vi "RESTORE USER TO DATABASE.vi"(10 "DATA IN":string[][](array[string]), 11 "REFERENCES":T1) -> ()   [LabVIEW 2019]
uses:
  Controls/References Cluster.ctl
  Controls/Custom Calendar/Custom Calendar.xctl
  Controls/Table Data Types/User Archive Data Type.ctl
  Controls/Table Data Types/User Data Type.ctl
  <vilib>/addons/database/Connection.llb/DB Tools Open Connec (String).vi
  <vilib>/addons/database/_DB Variant To Data/Database Variant To Data.xnode
  <vilib>/addons/database/NI_Database_API.lvlib
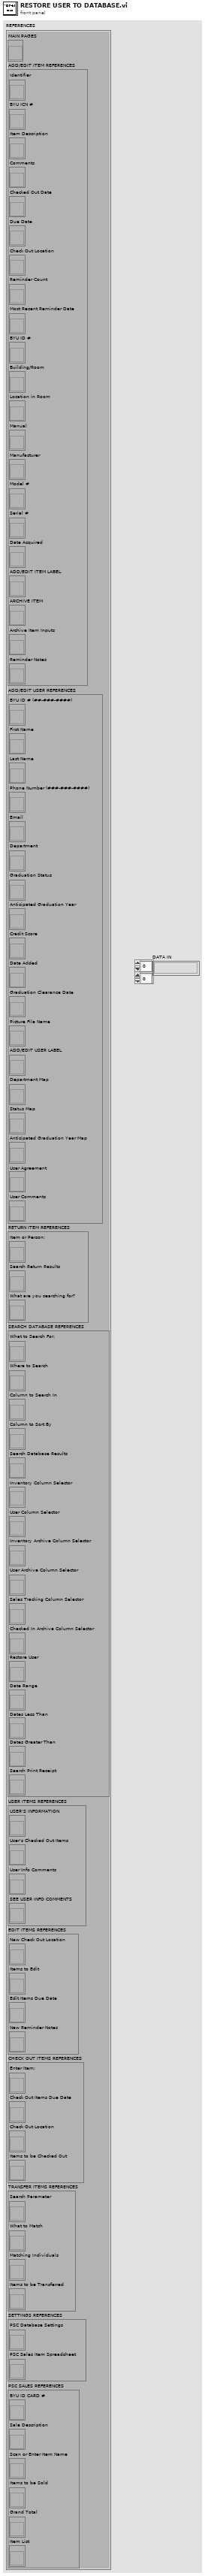
[diagram p1: front panel]
types:
  T1 = typedef "References Cluster.ctl" = cluster{"MAIN PAGES":refnum<vi>, "ADD/EDIT ITEM REFERENCES":cluster{"Identifier":refnum<vi>, "BYU ICN #":refnum<vi>, "Item Description":refnum<vi>, "Comments":refnum<vi>, "Checked Out Date":refnum<vi>, "Due Date":refnum<vi>, "Check Out Location":refnum<vi>, "Reminder Count":refnum<vi>, "Most Recent Reminder Date":refnum<vi>, "BYU ID #":refnum<vi>, "Building/Room":refnum<vi>, "Location in Room":refnum<vi>, "Manual":refnum<vi>, "Manufacturer":refnum<vi>, "Model #":refnum<vi>, "Serial #":refnum<vi>, "Date Acquired":refnum<vi>, "ADD/EDIT ITEM LABEL":refnum<vi>, "ARCHIVE ITEM":refnum<vi>, "Archive Item Inputs":refnum<vi>, "Reminder Notes":refnum<vi>}, "ADD/EDIT USER REFERENCES":cluster{"BYU ID # (##-###-####)":refnum<vi>, "First Name":refnum<vi>, "Last Name":refnum<vi>, "Phone Number (###-###-####)":refnum<vi>, "Email":refnum<vi>, "Department":refnum<vi>, "Graduation Status":refnum<vi>, "Anticipated Graduation Year":refnum<vi>, "Credit Score":refnum<vi>, "Date Added":refnum<vi>, "Graduation Clearance Date":refnum<vi>, "Picture File Name":refnum<vi>, "ADD/EDIT USER LABEL":refnum<vi>, "Department Map":refnum<vi>, "Status Map":refnum<vi>, "Anticipated Graduation Year Map":refnum<vi>, "User Agreement":refnum<vi>, "User Comments":refnum<vi>}, "RETURN ITEM REFERENCES":cluster{"Item or Person:":refnum<vi>, "Search Return Results":refnum<vi>, "What are you searching for?":refnum<vi>}, "SEARCH DATABASE REFERENCES":cluster{"What to Search For:":refnum<vi>, "Where to Search":refnum<vi>, "Column to Search In":refnum<vi>, "Column to Sort By":refnum<vi>, "Search Database Results":refnum<vi>, "Inventory Column Selector":refnum<vi>, "User Column Selector":refnum<vi>, "Inventory Archive Column Selector":refnum<vi>, "User Archive Column Selector":refnum<vi>, "Sales Tracking Column Selector":refnum<vi>, "Checked In Archive Column Selector":refnum<vi>, "Restore User":refnum<vi>, "Date Range":refnum<vi>, "Dates Less Than":refnum<vi>, "Dates Greater Than":refnum<vi>, "Search Print Receipt":refnum<vi>}, "USER ITEMS REFERENCES":cluster{"USER'S INFORMATION":refnum<vi>, "User's Checked Out Items":refnum<vi>, "User Info Comments":refnum<vi>, "SEE USER INFO COMMENTS":refnum<vi>}, "EDIT ITEMS REFERENCES":cluster{"New Check Out Location":refnum<vi>, "Items to Edit":refnum<vi>, "Edit Items Due Date":refnum<vi>, "New Reminder Notes":refnum<vi>}, "CHECK OUT ITEMS REFERENCES":cluster{"Enter Item:":refnum<vi>, "Check Out Items Due Date":refnum<vi>, "Check Out Location":refnum<vi>, "Items to be Checked Out":refnum<vi>}, "TRANSFER ITEMS REFERENCES":cluster{"Search Parameter":refnum<vi>, "What to Match":refnum<vi>, "Matching Individuals":refnum<vi>, "Items to be Transferred":refnum<vi>}, "SETTINGS REFERENCES":cluster{"PSC Database Settings":refnum<vi>, "PSC Sales Item Spreadsheet":refnum<vi>}, "PSC SALES REFERENCES":cluster{"BYU ID CARD #":refnum<vi>, "Sale Description":refnum<vi>, "Scan or Enter Item Name":refnum<vi>, "Items to be Sold":refnum<vi>, "Grand Total":refnum<vi>, "Item List":refnum<vi>}}
  T2 = cluster{"What to Search For:":refnum<vi>, "Where to Search":refnum<vi>, "Column to Search In":refnum<vi>, "Column to Sort By":refnum<vi>, "Search Database Results":refnum<vi>, "Inventory Column Selector":refnum<vi>, "User Column Selector":refnum<vi>, "Inventory Archive Column Selector":refnum<vi>, "User Archive Column Selector":refnum<vi>, "Sales Tracking Column Selector":refnum<vi>, "Checked In Archive Column Selector":refnum<vi>, "Restore User":refnum<vi>, "Date Range":refnum<vi>, "Dates Less Than":refnum<vi>, "Dates Greater Than":refnum<vi>, "Search Print Receipt":refnum<vi>}
  T3 = typedef "User Data Type.ctl" = cluster{"BYU ID #":string, "First Name":string, "Last Name":string, "Phone Number":string, "Email":string, "Department":string, "Graduation Status":string, "Anticipated Graduation Year":string, "Credit Score":dbl, "Date Added":string, "Graduation Clearance Date":string, "Picture File Name":string, "User Comments":string}
  T4 = typedef "User Archive Data Type.ctl" = cluster{"BYU ID #":string, "First Name":string, "Last Name":string, "Phone Number":string, "Email":string, "Department":string, "Graduation Status":string, "Anticipated Graduation Year":string, "Credit Score":dbl, "Date Added":string, "Graduation Clearance Date":string, "Picture File Name":string, "Date Archived":string}
  T5 = typedef "NI_Database_API.lvlib/Conn ObjectReference.ctl" = refnum<k1>
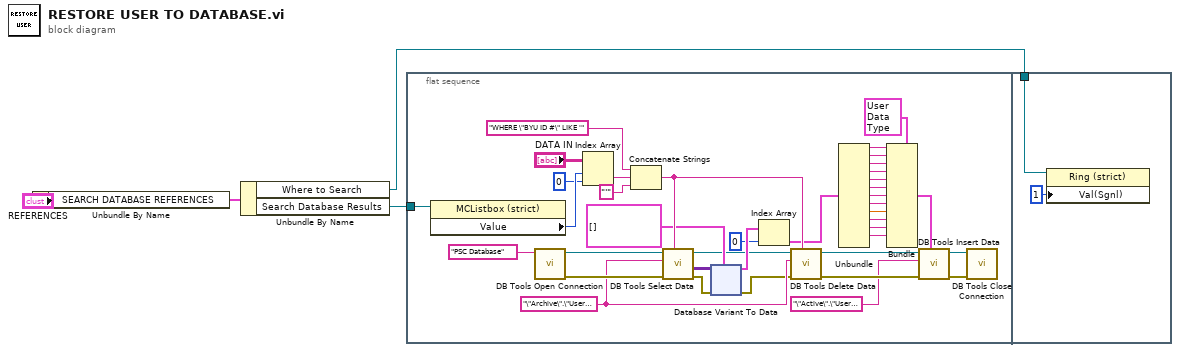
[diagram p0: block diagram]
diagram:
  n1 = Unbundle By Name("REFERENCES") -> ("SEARCH DATABASE REFERENCES"=w3:T2)
  n2 = Unbundle By Name(w3) -> ("Where to Search"=w1:refnum<vi>, "Search Database Results"=w2:refnum<vi>)
  n3 = flat-sequence {
    tunnel: w2 -> [w43]
    tunnel: w1 -> [w458]
    frame #0 {
      w32 = "\"Archive\".\"Users\""
      n4 = property class="MCListbox (strict)"(reference=w43) -> ("Value"=w41:i32)  [unwired: 1 in, 2 out]
      n5 = call-poly <vilib>:"DB Tools Open Connection.vi"("connection information"="PSC Database") -> ("error out"=w35:errorcluster, "connection reference"=w34:T5)  [unwired: 7 in]
      n6 = Index Array(array="DATA IN", index (row)=w41, index (col)=0 ("disabled index (col)")) -> (element=w37:string)
      n7 = Concatenate Strings("WHERE \"BYU ID #\" LIKE '", w37, "'") -> (w33:string)
      n8 = call <vilib>:"DB Tools Select Data.vi"("condition"=w33, "error in (no error)"=w35, "table"=w32, "connection reference"=w34) -> ("error out"=w31:errorcluster, "data"=w30:variant[][], "connection reference out"=w26:T5)  [unwired: 2 in]
      n9 = xnode "Database Variant To Data"("database variant"=w30, "error in (no error)"=w31, "type"=T4[] []) -> ("data"=w28:T4[], "error out"=w25:errorcluster)
      n10 = Index Array(array=w28, index=0) -> (element=w24:T4)
      n11 = call <vilib>:"DB Tools Delete Data.vi"("condition"=w33, "error in (no error)"=w25, "table"=w32, "connection reference"=w26) -> ("error out"=w8:errorcluster, "connection reference out"=w9:T5)  [unwired: 6 in]
      n12 = Unbundle(w24) -> ("BYU ID #"=w22:string, "First Name"=w21:string, "Last Name"=w20:string, "Phone Number"=w19:string, "Email"=w18:string, "Department"=w17:string, "Graduation Status"=w16:string, "Anticipated Graduation Year"=w14:string, "Credit Score"=w15:dbl, "Date Added"=w13:string, "Graduation Clearance Date"=w12:string, "Picture File Name"=w11:string)  [unwired: 1 out]
      n13 = Bundle(cluster=T3 {"BYU ID #"="", "First Name"="", "Last Name"="", "Phone Number"="", "Email"="", "Department"="", "Graduation Status"="", "Anticipated Graduation Year"="", "Credit Score"=0.0, "Date Added"="", "Graduation Clearance Date"="", "Picture File Name"="", "User Comments"=""} ("USER DATA TYPE"), "BYU ID #"=w22, "First Name"=w21, "Last Name"=w20, "Phone Number"=w19, "Email"=w18, "Department"=w17, "Graduation Status"=w16, "Anticipated Graduation Year"=w14, "Credit Score"=w15, "Date Added"=w13, "Graduation Clearance Date"=w12, "Picture File Name"=w11) -> (w10:T3)  [unwired: 1 in]
      n14 = call <vilib>:"DB Tools Insert Data.vi"("data"=w10, "error in (no error)"=w8, "table"="\"Active\".\"Users\"", "connection reference"=w9) -> ("error out"=w6:errorcluster, "connection reference out"=w5:T5)  [unwired: 6 in]
      n15 = call <vilib>:"DB Tools Close Connection.vi"("error in (no error)"=w6, "connection reference"=w5) -> ()  [unwired: 5 in, 1 out]
    }
    frame #1 {
      n16 = property class="Ring (strict)"(reference=w458, "Val(Sgnl)"=u16 1 ("Value (Signaling)")) -> ()  [unwired: 1 in, 2 out]
    }
  }
